vi "AnalysatorNameEindeutig.vi"(10 "AnalysatorDefinition":T1, 11 "AnalysatorListe":T1[](array[typedef])) -> (0 "unique":bool, 1 "Index":i32, 2 "AnalysatorDefinition out":T1, 3 "AnalysatorListe out":T1[](array[typedef]))   [LabVIEW 2020, in "System Einstellungen V2.lvlib"]
uses:
  System Einstellungen V2.lvlib
  AnalysatorDefinition.ctl
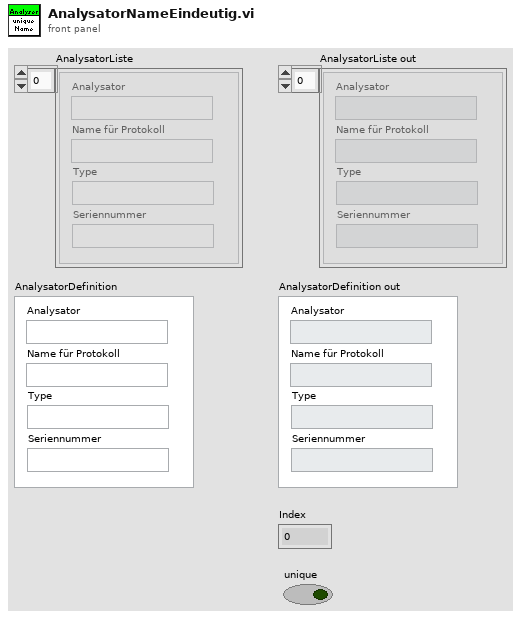
[diagram p1: front panel]
types:
  T1 = typedef "System Einstellungen V2.lvlib/AnalysatorDefinition.ctl" = cluster{"Analysator":string, "Name für Protokoll":string, "Type":string, "Seriennummer":string}
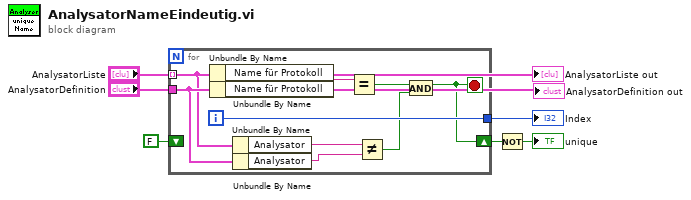
[diagram p0: block diagram]
diagram:
  n1 = for {
    tunnel: "AnalysatorDefinition" -> [w9]
    tunnel: "AnalysatorListe" -> [w10] mode=indexing
    tunnel: [w14] -> w5
    shift-right: [w13] -> w2
    shift-left: FALSE -> [_]
    i -> [w14]
    stop <- w13 stop-if-true
    n2 = Unbundle By Name(w10) -> ("Name für Protokoll"=w16:string)
    n3 = Unbundle By Name(w9) -> ("Name für Protokoll"=w15:string)
    n4 = Unbundle By Name(w10) -> ("Analysator"=w8:string)
    n5 = Unbundle By Name(w9) -> ("Analysator"=w7:string)
    n6 = Equal?(x=w16, y=w15) -> (x = y?=w12:bool)
    n7 = Not Equal?(x=w8, y=w7) -> (x != y?=w11:bool)
    n8 = And(x=w12, y=w11) -> (x .and. y?=w13:bool)
  }
  "Index" <- w5
  n9 = Not(x=w2) -> (.not. x?=→"unique":bool)
  "AnalysatorListe out" <- "AnalysatorListe"
  "AnalysatorDefinition out" <- "AnalysatorDefinition"
